vi "PH_VacuumControl.Get Unit.vi"(0 "i ref in":refnum<vi>, 5 "error in (no error)":errorcluster) -> (14 "i ref out":refnum<vi>, 19 "error out":errorcluster)   [LabVIEW 2014, in "PH_VacuumControl.lvlib"]
doc: "This VI asks the vacuum gauge for the current unit and sets it to own attributes and manipulates several GUI elements."
uses:
  PH_VacuumControl.lvlib
  instr.lib/AGCxxx/AGCxxx - Driver.lvlib
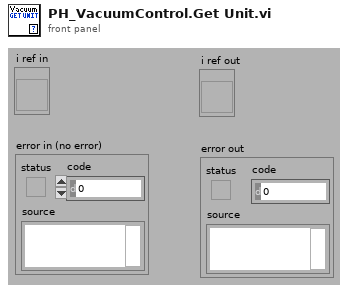
[diagram p1: front panel]
types:
  T1 = typedef "PH_VacuumControl.lvlib/PH_VacuumControl.i attribute.ctl" = cluster{"GUI Refs":cluster{"Exit":refnum<vi>, "Set Unit":refnum<vi>, "Device found":refnum<vi>, "Busy":refnum<vi>, "State":refnum<vi>, "Delete":refnum<vi>, "Channels":refnum<vi>, "Channel Name":refnum<vi>, "Trend":refnum<vi>, "Logarithmic":refnum<vi>, "Limit reached":refnum<vi>, "Channel Name 1 MT":refnum<vi>, "Channel Name 2 MT":refnum<vi>, "Trend MT":refnum<vi>, "Logarithmic MT":refnum<vi>, "Limit reached MT":refnum<vi>}, "Device found":bool, "Busy":bool, "Selected Unit":i32, "Channels [mbar]":T2, "Channel Names":cluster{"Channel 1":string, "Channel 2":string, "Channel 3":string, "Channel 4":string, "Channel 5":string, "Channel 6":string}, "Status":T3, "AGCxxx VISA Cluster":T4, "Instr Firmware Revision":string, "Service IDs Pressure":cluster{"Channel 1":i32, "Channel 2":i32, "Channel 3":i32, "Channel 4":i32, "Channel 5":i32, "Channel 6":i32}, "Service IDs Limits":cluster{"Channel 1":i32, "Channel 2":i32, "Channel 3":i32, "Channel 4":i32, "Channel 5":i32, "Channel 6":i32}, "Trend":cluster{"Start Point":timestamp, "Pressures [mbar] Channel 1":dbl[], "Pressures [mbar] Channel 2":dbl[], "Pressures [mbar] Channel 3":dbl[], "Pressures [mbar] Channel 4":dbl[], "Pressures [mbar] Channel 5":dbl[], "Pressures [mbar] Channel 6":dbl[], "Timebase [s]":i32[], "Trend Channel":u16, "Start Fit":dbl, "Trend Channel 1 MT":u16, "Trend Channel 2 MT":u16, "Start or continue Fit MT":dbl, "Continue or start Fit MT":dbl, "Datasets strored":i32, "Dataarray Size":i32}, "Running":bool}
  T2 = typedef "PH_VacuumControl.lvlib/PH_VacuumControl.Channels.ctl" = cluster{"Channel 1":dbl, "Channel 2":dbl, "Channel 3":dbl, "Channel 4":dbl, "Channel 5":dbl, "Channel 6":dbl, "Name Channel 1":string, "Name Channel 2":string, "Name Channel 3":string, "Name Channel 4":string, "Name Channel 5":string, "Name Channel 6":string, "Upper Limit":dbl, "Upper Limit 2":dbl, "Upper Limit 3":dbl, "Upper Limit 4":dbl, "Upper Limit 5":dbl, "Upper Limit 6":dbl}
  T3 = typedef "PH_StatusHandler.lvlib/PH_StatusHandler.Status.ctl" = i16
  T4 = typedef "AGCxxx - Driver.lvlib/AGCxxx VISA Control.ctl" = cluster{"VISA resource name":refnum<visa-resource-name>, "VISA Timeout Value (1000 ms)":u32, "Lock Timeout (1000 ms)":u32, "MAX Channel (6)":i32}
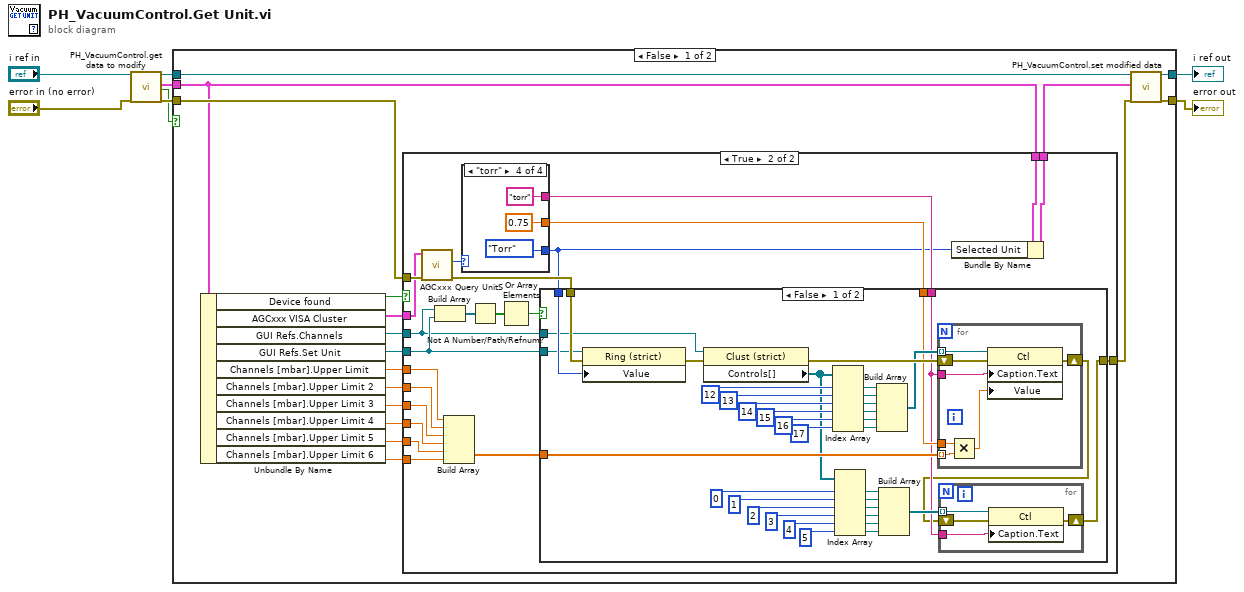
[diagram p0: block diagram]
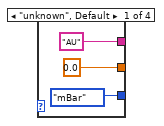
[diagram p4: hidden frame]
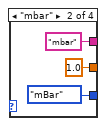
[diagram p5: hidden frame]
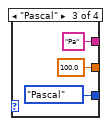
[diagram p6: hidden frame]
diagram:
  n1 = call "PH_VacuumControl.get data to modify.vi"("i ref in"="i ref in", "error in (no error)"="error in (no error)") -> ("i ref out"=w4:refnum<vi>, "i attribute"=w8:T1, "timed out"=w1:bool, "error out"=w6:errorcluster)  [unwired: 14 in]
  n2 = case shown="False" w1 {
    tunnel: w8 -> [w10 _]
    tunnel: w6 -> [w11 w112]
    tunnel: w4 -> [w15 w113]
    tunnel: [w14 w113] -> w3
    tunnel: [w13 w112] -> w2
    frame False {
      n3 = Unbundle By Name(w10) -> ("Device found"=w19:bool, "AGCxxx VISA Cluster"=w16:T4, "GUI Refs.Channels"=w18:refnum<vi>, "GUI Refs.Set Unit"=w17:refnum<vi>, "Channels [mbar].Upper Limit"=w20:dbl, "Channels [mbar].Upper Limit 2"=w21:dbl, "Channels [mbar].Upper Limit 3"=w22:dbl, "Channels [mbar].Upper Limit 4"=w23:dbl, "Channels [mbar].Upper Limit 5"=w24:dbl, "Channels [mbar].Upper Limit 6"=w25:dbl)
      n4 = case shown="True" w19 {
        tunnel: w11 -> [w27 w49]
        tunnel: w16 -> [_ w48]
        tunnel: [w27 w45] -> w12
        tunnel: w17 -> [_ w42]
        tunnel: w18 -> [_ w41]
        tunnel: w20 -> [_ w38]
        tunnel: w21 -> [_ w37]
        tunnel: w22 -> [_ w36]
        tunnel: w23 -> [_ w35]
        tunnel: w24 -> [_ w34]
        tunnel: w25 -> [_ w33]
        tunnel: w10 -> [w26 w30]
        tunnel: [w26 w28] -> w9
        frame False {
        }
        frame True {
          n5 = call "AGCxxx Query UnitS.vi"("error in (no error)"=w49, "AGCxxx VISA Cluster"=w48) -> ("error out"=w46:errorcluster, "unit"=w47:enum16{"unknown", "mbar", "Pascal", "torr"})  [unwired: 6 in, 2 out]
          n6 = Build Array(w41, w42) -> (w44:refnum<vi>[])
          n7 = Build Array(w38, w37, w36, w35, w34, w33) -> (w32:dbl[])
          n8 = case shown="\"torr\"" w47 {
            tunnel: ["AU" "mbar" "Pa" "torr"] -> w39
            tunnel: [enum16{"mBar", "Pascal", "Torr"}."mBar" ("Set Unit") enum16{"mBar", "Pascal", "Torr"}."mBar" ("Set Unit") enum16{"mBar", "Pascal", "Torr"}."Pascal" ("Set Unit") enum16{"mBar", "Pascal", "Torr"}."Torr" ("Set Unit")] -> w29
            tunnel: [0.0 ("x") 1.0 ("x") 100.0 ("x") 0.75 ("x")] -> w31
            frame "unknown", Default {
            }
            frame "mbar" {
            }
            frame "Pascal" {
            }
            frame "torr" {
            }
          }
          n9 = Not A Number/Path/Refnum?(number/path/refnum=w44) -> (NaN/Path/Refnum?=w43:bool[])
          n10 = Or Array Elements(Boolean array=w43) -> (logical OR=w40:bool)
          n11 = case shown="False" w40 {
            tunnel: w46 -> [w87 w99]
            tunnel: w29 -> [w86 _]
            tunnel: [w50 w99] -> w45
            tunnel: w42 -> [w84 _]
            tunnel: w41 -> [w83 _]
            tunnel: w39 -> [w52 _]
            tunnel: w32 -> [w68 _]
            tunnel: w31 -> [w67 _]
            frame False {
              n12 = property class="Ring (strict)"(reference=w84, error in=w87, "Value"=w86) -> (error out=w85:errorcluster)  [unwired: 1 out]
              n13 = property class="Clust (strict)"(reference=w83, error in=w85) -> (error out=w70:errorcluster, "Controls[]"=w55:refnum<vi>[])  [unwired: 1 out]
              n14 = Index Array(array=w55, index #1=12 ("index"), index #2=13 ("index"), index #3=14 ("index"), index #4=15 ("index"), index #5=16 ("index"), index #6=17 ("index")) -> (element #1=w76:refnum<vi>, element #2=w75:refnum<vi>, element #3=w74:refnum<vi>, element #4=w73:refnum<vi>, element #5=w72:refnum<vi>, element #6=w71:refnum<vi>)
              n15 = Index Array(array=w55, index #1=0 ("index"), index #2=1 ("index"), index #3=2 ("index"), index #4=3 ("index"), index #5=4 ("index"), index #6=5 ("index")) -> (element #1=w61:refnum<vi>, element #2=w60:refnum<vi>, element #3=w59:refnum<vi>, element #4=w58:refnum<vi>, element #5=w57:refnum<vi>, element #6=w56:refnum<vi>)
              n16 = Build Array(w76, w75, w74, w73, w72, w71) -> (w69:refnum<vi>[])
              n17 = Build Array(w61, w60, w59, w58, w57, w56) -> (w53:refnum<vi>[])
              n18 = for {
                shift-right: [w97] -> w51
                shift-left: w70 -> [w98]
                tunnel: w69 -> [w96] mode=indexing
                tunnel: w52 -> [w95]
                tunnel: w68 -> [w94] mode=indexing
                tunnel: w67 -> [w92]
                n19 = Multiply(x=w92, y=w94) -> (x*y=w93:dbl)
                n20 = property class="Ctl"(reference=w96, error in=w98, "Caption.Text"=w95, "Value"=w93) -> (error out=w97:errorcluster)  [unwired: 1 out]
              }
              n21 = for {
                shift-right: [w90] -> w50
                shift-left: w51 -> [w91]
                tunnel: w53 -> [w89] mode=indexing
                tunnel: w52 -> [w88]
                n22 = property class="Ctl"(reference=w89, error in=w91, "Caption.Text"=w88) -> (error out=w90:errorcluster)  [unwired: 1 out]
              }
            }
            frame True {
            }
          }
          n23 = Bundle By Name(cluster=w30, "Selected Unit"=w29) -> (w28:T1)
        }
      }
      n24 = call "PH_VacuumControl.set modified data.vi"("i ref in"=w15, "i attribute"=w9, "error in (no error)"=w12) -> ("i ref out"=w14:refnum<vi>, "error out"=w13:errorcluster)  [unwired: 15 in]
    }
    frame True {
    }
  }
  "error out" <- w2
  "i ref out" <- w3
